vi "stan 1.vi"() -> ()   [LabVIEW 2020]
panel:
  in  "error in (no error) 2":errorcluster
  out "error in (no error)":errorcluster
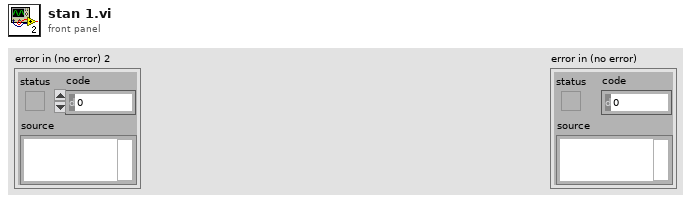
[diagram p1: front panel]
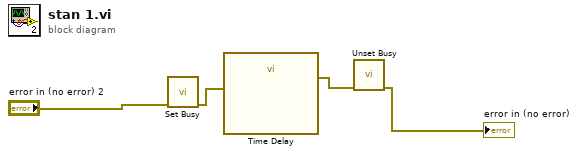
[diagram p0: block diagram]
diagram:
  n1 = call <vilib>:"Set Busy.vi"("error in (no error)"="error in (no error) 2") -> ("error out"=w3:errorcluster)  [unwired: 9 in, 1 out]
  n2 = call "Time Delay"("error in (no error)"=w3) -> ("error out"=w2:errorcluster)  [unwired: 10 in]
  n3 = call <vilib>:"Unset Busy.vi"("error in (no error)"=w2) -> ("error out"=→"error in (no error)":errorcluster)  [unwired: 10 in]
